vi "mqttFlagsWrite.vi"(0 "mqtt in":refnum<class "mqtt.lvclass">, 5 "connFlags":T1, 11 "error in (no error)":errorcluster) -> (4 "mqtt out":refnum<class "mqtt.lvclass">, 15 "error out":errorcluster)   [LabVIEW 2017, in "mqtt.lvclass"]
uses:
  mqtt.lvclass
  mqttTypedef/mqttConnectionFlags.ctl
  mqtt.lvclass/mqtt.ctl
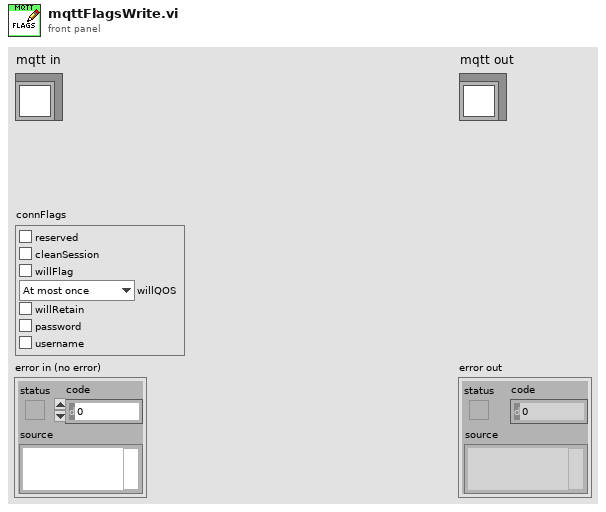
[diagram p1: front panel]
types:
  T1 = typedef "mqttConnectionFlags.ctl" = cluster{"reserved":bool, "clean session":bool, "will flag":bool, "willQOS":enum8{"At most once", "At least once", "Exactly once", "Reserved"}, "will retain":bool, "password":bool, "user name":bool}
  T2 = enum8{"At most once", "At least once", "Exactly once", "Reserved"}
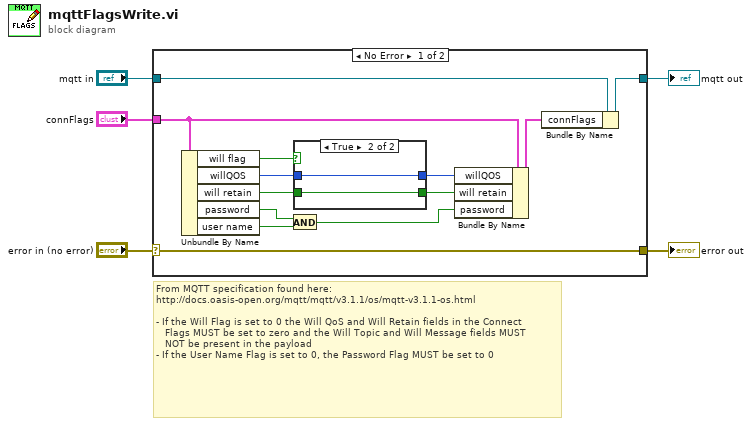
[diagram p0: block diagram]
diagram:
  # "From MQTT specification found here:\nhttp://docs.oasis-open.org/mqtt/mqtt/v3.1.1/os/mqtt-v3.1.1-os.html\n\n- If the Will Flag is set to 0 the Will QoS and Will Retain fields in the Connect\n   Flags MUST be set to zero and the Will Topic and Will Message fields MUST\n   NOT be present in the payload\n- If the User Name Flag is set to 0, the Password Flag MUST be set to 0"
  n1 = case shown="No Error" "error in (no error)" {
    selector: "error in (no error)" -> [w18 w21]
    tunnel: [w18 w21] -> w4
    tunnel: [w16 w22] -> w2
    tunnel: "mqtt in" -> [w17 w22]
    tunnel: "connFlags" -> [w15 _]
    frame No Error {
      n2 = Unbundle By Name(w15) -> ("will flag"=w13:bool, "willQOS"=w11:T2, "will retain"=w9:bool, "password"=w8:bool, "user name"=w7:bool)
      n3 = And(x=w8, y=w7) -> (x .and. y?=w6:bool)
      n4 = case shown="True" w13 {
        tunnel: [_ w20] -> w12
        tunnel: w11 -> [_ w20]
        tunnel: [_ w19] -> w10
        tunnel: w9 -> [_ w19]
        frame False {
        }
        frame True {
        }
      }
      n5 = Bundle By Name(cluster=w15, "willQOS"=w12, "will retain"=w10, "password"=w6) -> (w14:T1)
      n6 = Bundle By Name(cluster=w17, "connFlags"=w14) -> (w16:refnum<class "mqtt.lvclass">)
    }
    frame Error {
    }
  }
  "error out" <- w4
  "mqtt out" <- w2
